vi "Detach MainPane.vi"(8 "error in (no error)":errorcluster, 11 "DemoMain in":refnum<class "DemoMain.lvclass">) -> (0 "error out":errorcluster, 3 "DemoMain out":refnum<class "DemoMain.lvclass">)   [LabVIEW 2012, in "Win8uiDemo.lvlib" / "DemoMain.lvclass"]
uses:
  DemoMain.lvclass
  <vilib>/ActorFramework/Message Enqueuer/Message Enqueuer.lvclass
  Win8uiFramework/MainController.lvclass/MainController.ctl
  <vilib>/ActorFramework/Message Enqueuer/Message Enqueuer.lvclass/Message Enqueuer.ctl
  Win8uiFramework/Read MainPane Enqueuer.vi
  Win8uiFramework/Write MainPane Enqueuer.vi
  <vilib>/ActorFramework/Message Enqueuer/Enqueue.vi
  <vilib>/ActorFramework/Message Priority Queue/Priority Enqueue.vi
  Win8uiFramework/Remove From SubPanel Msg.lvclass
  Win8uiFramework/ViewableActor Messages/Open Front Panel Msg/Open Front Panel Msg.lvclass
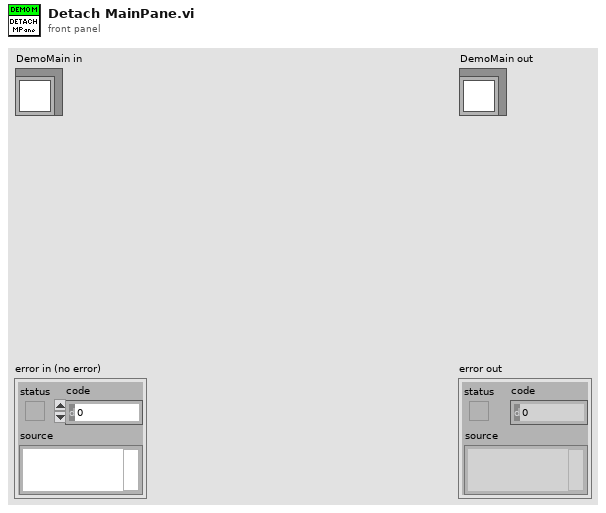
[diagram p1: front panel]
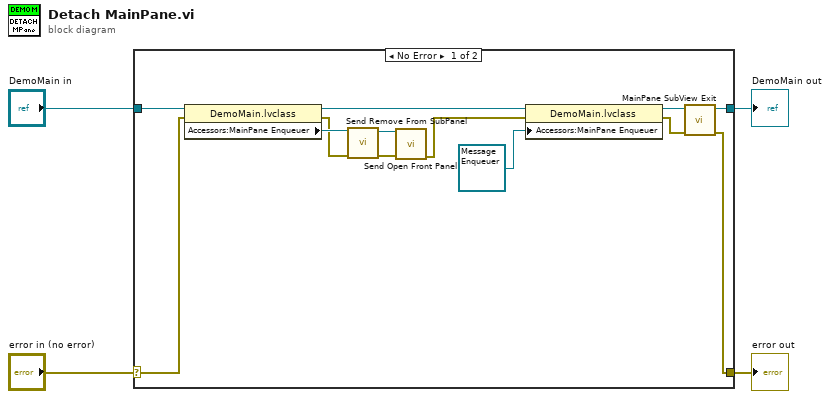
[diagram p0: block diagram]
diagram:
  n1 = case shown="No Error" "error in (no error)" {
    selector: "error in (no error)" -> [w7 w19]
    tunnel: [w6 w19] -> w3
    tunnel: [w13 w18] -> w1
    tunnel: "DemoMain in" -> [w17 w18]
    frame No Error {
      n2 = property class="DemoMain.lvclass"(reference=w17, error in=w7) -> (reference out=w14:refnum<class "DemoMain.lvclass">, error out=w12:errorcluster, "Accessors:MainPane Enqueuer"=w16:refnum<class "Message Enqueuer.lvclass">)
      n3 = call "Send Remove From SubPanel.vi"("error in (no error)"=w12, "Message Enqueuer"=w16) -> ("error out"=w11:errorcluster, "Message Enqueuer out"=w15:refnum<class "Message Enqueuer.lvclass">)  [unwired: 8 in]
      n4 = call "Send Open Front Panel.vi"("error in (no error)"=w11, "Message Enqueuer"=w15) -> ("error out"=w9:errorcluster)  [unwired: 8 in, 1 out]
      n5 = property class="DemoMain.lvclass"(reference=w14, error in=w9, "Accessors:MainPane Enqueuer"=refnum<class "Message Enqueuer.lvclass"> refnum ("MainPane Enqueuer")) -> (reference out=w10:refnum<class "DemoMain.lvclass">, error out=w8:errorcluster)
      n6 = call-dynamic "MainPane SubView Exit.vi"("error in (no error)"=w8, "MainController in"=w10) -> ("error out"=w6:errorcluster, "MainController out"=w13:refnum<class "DemoMain.lvclass">)  [unwired: 8 in]
    }
    frame Error {
    }
  }
  "error out" <- w3
  "DemoMain out" <- w1
